vi "Close Error Log.vi"(8 "Error In":errorcluster) -> (0 "Error Out":errorcluster)   [LabVIEW 2016, in "Error Manager.lvlib" / "Error Log.lvclass"]
doc: "This VI closes the reference to the Error Log file."
uses:
  Error Log.lvclass
  Error Log Ref (class variable).vi
panel:
  # "Input\nInputs to the VI"
  # "Development\nControls or indicators that are useful for development or testing, but which are not outputs of the VI."
  # "Output\nOutputs of the VI"
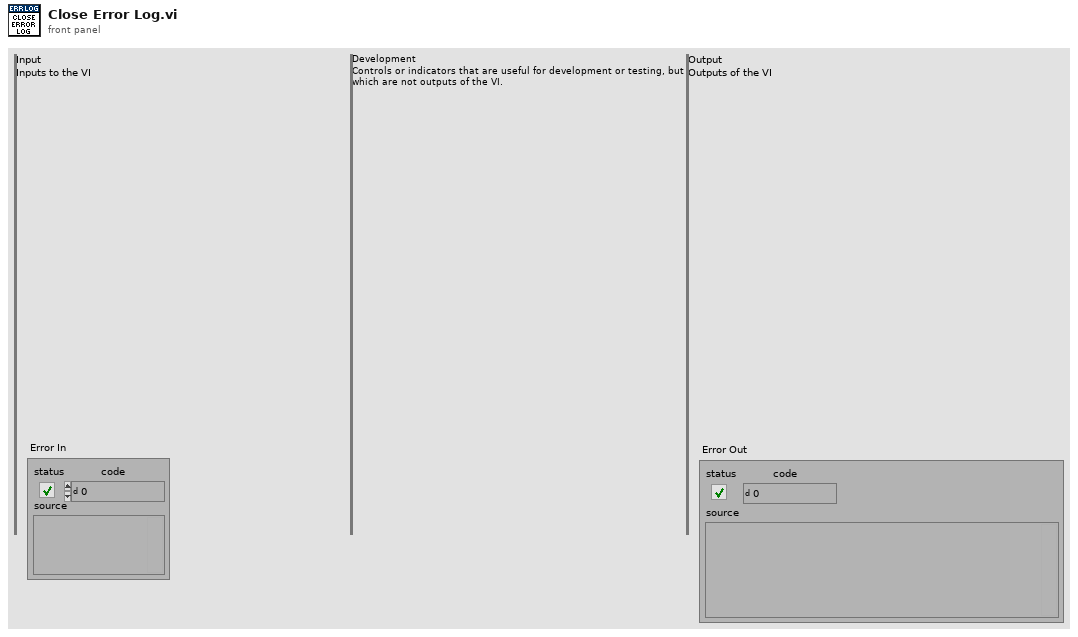
[diagram p1: front panel]
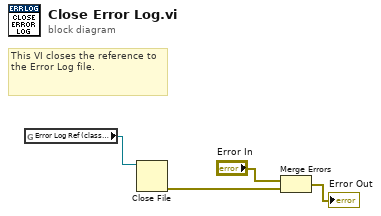
[diagram p0: block diagram]
diagram:
  # "This VI closes the reference to the Error Log file."
  n1 = global read "Error Log Ref (class variable).vi" item#0() -> (w3:refnum<file>)
  n2 = Close File(refnum=w3) -> (error out=w4:errorcluster)  [unwired: 1 in, 1 out]
  n3 = Merge Errors("Error In", w4) -> (→"Error Out":errorcluster)
